vi "ReadPosition.vi"(0 "object in":refnum<class "Prior_Zmotor.lvclass">, 5 "error in (no error)":errorcluster) -> (14 "object out":refnum<class "Prior_Zmotor.lvclass">, 16 "Position (um)":dbl, 19 "error out":errorcluster)   [LabVIEW 2021, in "Prior_Zmotor.lvclass"]
uses:
  Prior_Zmotor.lvclass
  Prior_Zmotor.lvclass/Prior_Zmotor.ctl
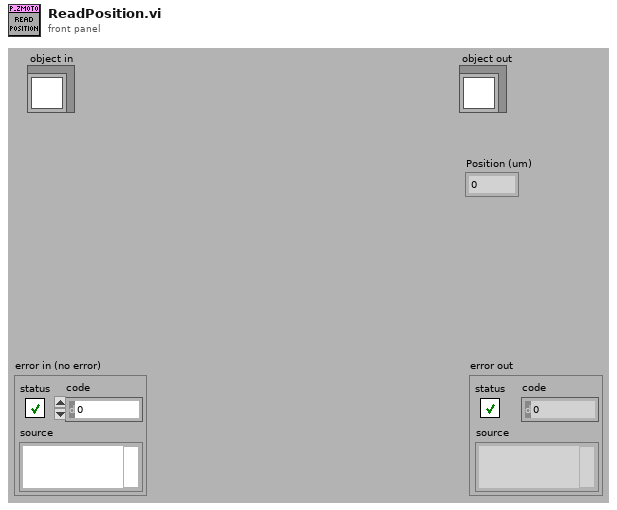
[diagram p1: front panel]
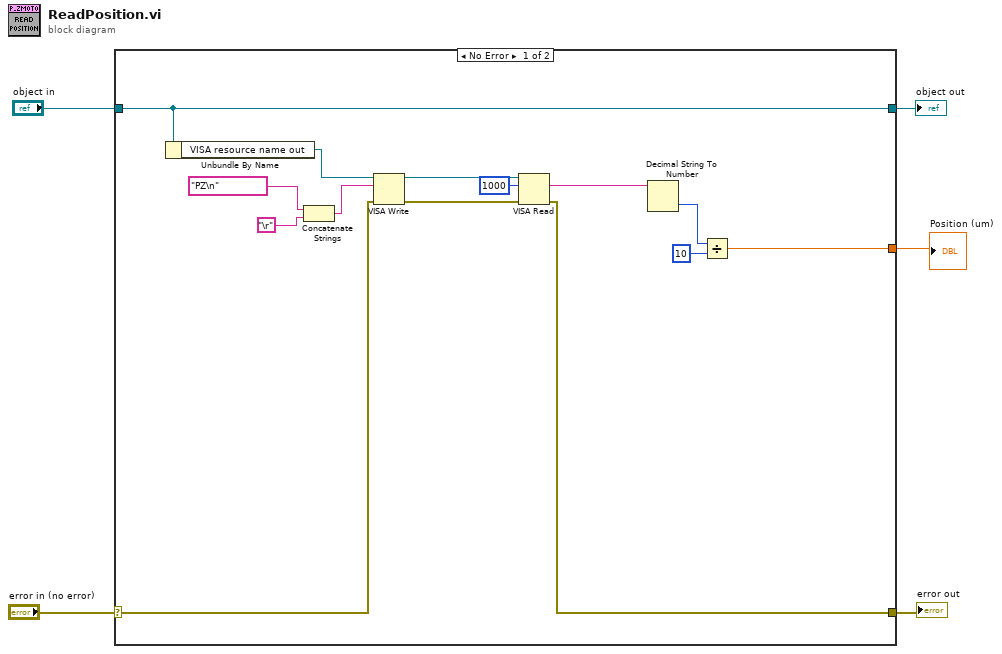
[diagram p0: block diagram]
diagram:
  n1 = case shown="No Error" "error in (no error)" {
    selector: "error in (no error)" -> [w15 w21]
    tunnel: [w14 w21] -> w4
    tunnel: [w19 w20] -> w2
    tunnel: "object in" -> [w19 w20]
    tunnel: [w10 _] -> w1
    frame No Error {
      n2 = Unbundle By Name(w19) -> ("VISA resource name out"=w18:refnum<visa-resource-name>)
      n3 = Concatenate Strings("PZ\n" ("write buffer"), "\r") -> (w8:string)
      n4 = VISA Write(VISA resource name=w18, write buffer=w8, error in (no error)=w15) -> (VISA resource name out=w17:refnum<visa-resource-name>, error out=w16:errorcluster)  [unwired: 1 out]
      n5 = VISA Read(VISA resource name=w17, byte count=u32 1000, error in (no error)=w16) -> (read buffer=w13:string, error out=w14:errorcluster)  [unwired: 2 out]
      n6 = Decimal String To Number(string=w13) -> (number=w12:i32)  [unwired: 2 in, 1 out]
      n7 = Divide(x=w12, y=10) -> (x/y=w10:dbl)
    }
    frame Error {
    }
  }
  "error out" <- w4
  "object out" <- w2
  "Position (um)" <- w1
